vi "Example.vi"() -> ()   [LabVIEW 2015]
uses:
  Drag & Drop New Multi.vi
  Drag & Drop Run Multi.vi
  Drag & Drop End Multi.vi
panel:
  out "Waveform Chart":dbl(graph)
  out "Boolean":bool
  in  "stop":bool
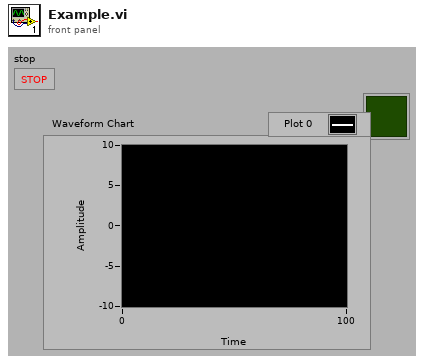
[diagram p1: front panel]
types:
  T1 = cluster{"Event Registration Refnum":refnum<event-registration>, "Ctl Refnum":refnum<vi>}[]
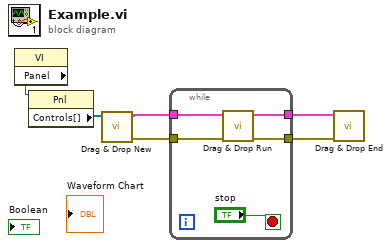
[diagram p0: block diagram]
diagram:
  n1 = property class="VI"() -> ("Panel"=w2:refnum<vi>)  [unwired: 2 in, 2 out]
  n2 = property class="Pnl"(reference=w2) -> ("Controls[]"=w1:refnum<vi>[])  [unwired: 1 in, 2 out]
  n3 = call-poly "Drag & Drop New.vi"("References In"=w1) -> ("References Out"=w4:T1, "error out"=w3:errorcluster)  [unwired: 8 in]
  n4 = while {
    tunnel: w4 -> [w8]
    tunnel: [w7] -> w5
    tunnel: w3 -> [w10]
    tunnel: [w9] -> w6
    stop <- "stop" stop-if-true
    n5 = call-poly "Drag & Drop Run.vi"("References In"=w8, "error in"=w10) -> ("References Out"=w7:T1, "error out"=w9:errorcluster)  [unwired: 6 in]
  }
  n6 = call-poly "Drag & Drop End.vi"("errorin"=w6, "References In"=w5) -> ()  [unwired: 9 in, 1 out]
